vi "Unsubscribe.vi"(8 "error in (no error)":errorcluster, 10 "Subscriber Enq":refnum<class "Message Enqueuer.lvclass">, 11 "Publisher Actor in":refnum<class "Publisher Actor.lvclass">) -> (0 "error out":errorcluster, 3 "Publisher Actor out":refnum<class "Publisher Actor.lvclass">)   [LabVIEW 2021, in "Publisher Actor.lvclass"]
uses:
  Publisher Actor.lvclass
  Publisher Actor.lvclass/Publisher Actor.ctl
  6be3ff21-4fbc-4d31-91ed-3e2bd578510d.vi
  <vilib>/ActorFramework/Message Enqueuer/Message Enqueuer.lvclass
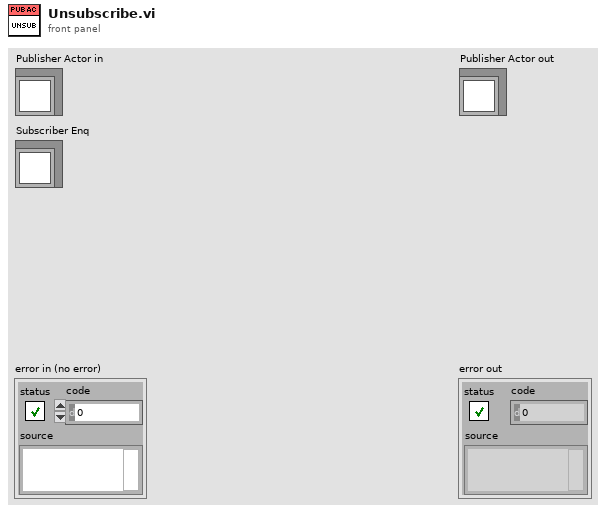
[diagram p1: front panel]
types:
  T1 = typedef "Context.ctl" = cluster{"Topic":string, "Source":string}
  T2 = map{T1, set{refnum<class "Message Enqueuer.lvclass">}}
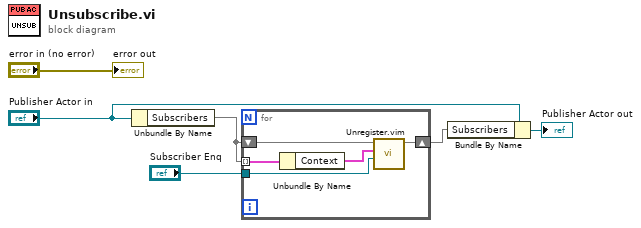
[diagram p0: block diagram]
diagram:
  n1 = Unbundle By Name("Publisher Actor in") -> ("Subscribers"=w5:T2)
  n2 = for {
    tunnel: w5 -> [w11] mode=indexing
    shift-right: [w7] -> w6
    shift-left: w5 -> [w9]
    tunnel: "Subscriber Enq" -> [w8]
    n3 = Unbundle By Name(w11) -> ("Context"=w10:T1)
    n4 = call "Unregister.vim"("set element"=w8, "key"=w10, "map in"=w9) -> ("map out"=w7:T2)  [unwired: 6 in, 2 out]
  }
  n5 = Bundle By Name(cluster="Publisher Actor in", "Subscribers"=w6) -> (→"Publisher Actor out":refnum<class "Publisher Actor.lvclass">)
  "error out" <- "error in (no error)"
